vi "Szybka_puste tablice.vi"(7 "Reset":bool, 8 "error in (no error)":errorcluster, 9 "Bufor in":T1, 11 "Kanaly in":T1) -> (0 "error out":errorcluster, 1 "Kanaly out":T1)   [LabVIEW 2013]
doc: "Use this template to build a VI to use as a subVI."
uses:
  Kontrolki/Przetwarzanie/Kanaly.ctl
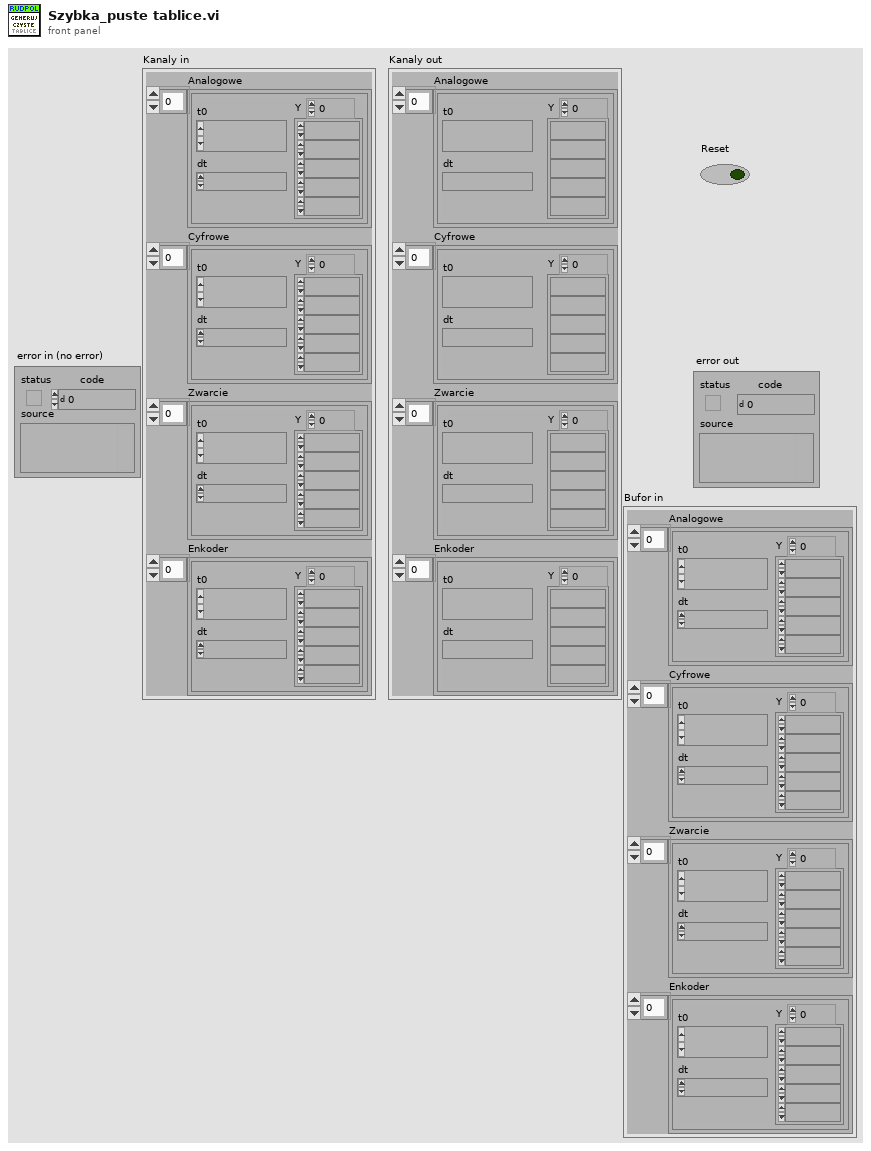
[diagram p1: front panel]
types:
  T1 = typedef "Kanaly.ctl" = cluster{"Analogowe":waveform(dbl)[], "Cyfrowe":waveform(dbl)[], "Zwarcie":waveform(dbl)[], "Enkoder":waveform(dbl)[]}
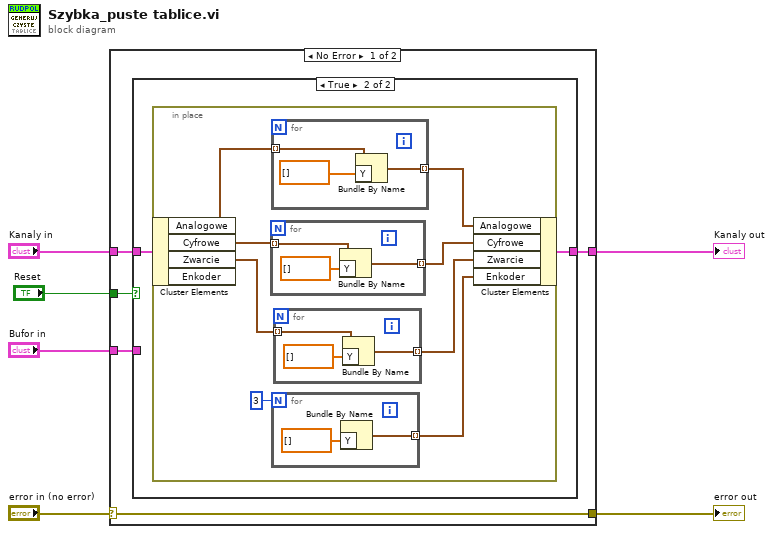
[diagram p0: block diagram]
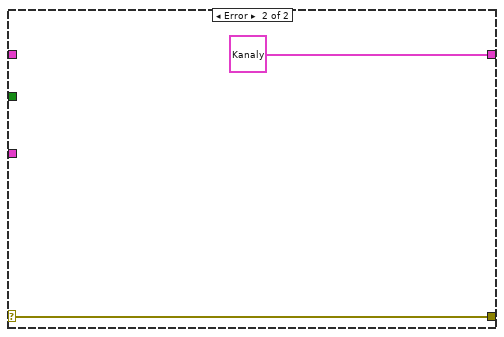
[diagram p3: hidden frame]
diagram:
  n1 = case shown="No Error" "error in (no error)" {
    selector: "error in (no error)" -> [w11 w35]
    tunnel: [w11 w35] -> w5
    tunnel: "Kanaly in" -> [w10 _]
    tunnel: [w9 T1 data[32432B] ("Kanaly in")] -> w3
    tunnel: "Bufor in" -> [w8 _]
    tunnel: "Reset" -> [w7 _]
    frame No Error {
      n2 = case shown="True" w7 {
        tunnel: w10 -> [_ w14]
        tunnel: [w12 w13] -> w9
        tunnel: w8 -> [w12 _]
        frame False {
        }
        frame True {
          n3 = in-place {
            n4 = in-place-cluster #1(w14) -> ("Analogowe"=w22:waveform(dbl)[], "Cyfrowe"=w21:waveform(dbl)[], "Zwarcie"=w20:waveform(dbl)[])  [unwired: 1 out]
            n5 = for {
              tunnel: w21 -> [w30] mode=indexing
              tunnel: [w28] -> w18 mode=indexing
              n6 = Bundle By Name(cluster=w30, "Y"=dbl[] []) -> (w28:waveform(dbl))
            }
            n7 = for {
              tunnel: [w32] -> w19 mode=indexing
              tunnel: w22 -> [w31] mode=indexing
              n8 = Bundle By Name(cluster=w31, "Y"=dbl[] []) -> (w32:waveform(dbl))
            }
            n9 = for {
              N: 3 -> [_]
              tunnel: [w23] -> w16 mode=indexing
              n10 = Bundle By Name("Y"=dbl[] []) -> (w23:waveform(dbl))  [unwired: 1 in]
            }
            n11 = for {
              tunnel: w20 -> [w27] mode=indexing
              tunnel: [w25] -> w17 mode=indexing
              n12 = Bundle By Name(cluster=w27, "Y"=dbl[] []) -> (w25:waveform(dbl))
            }
            n13 = in-place-cluster #1("Analogowe"=w19, "Cyfrowe"=w18, "Zwarcie"=w17, "Enkoder"=w16) -> (w13:T1)
          }
        }
      }
    }
    frame Error {
    }
  }
  "error out" <- w5
  "Kanaly out" <- w3
